vi "data read.vi"(8 "error in (no error)":errorcluster, 9 "新元素/子数组":u32, 10 "Array":u8[](array[numeric]), 11 "connection ID":refnum<k5>) -> (0 "error out":errorcluster, 1 "connection ID 2":refnum<k5>, 2 "数组 2":i32[][](array[numeric]), 3 "SEU number":u32)   [LabVIEW 2015]
panel:
  out "布尔":bool
  out "SEU？":bool
  in  "行":u32
  in  "停止":bool
  out "数据输出":string
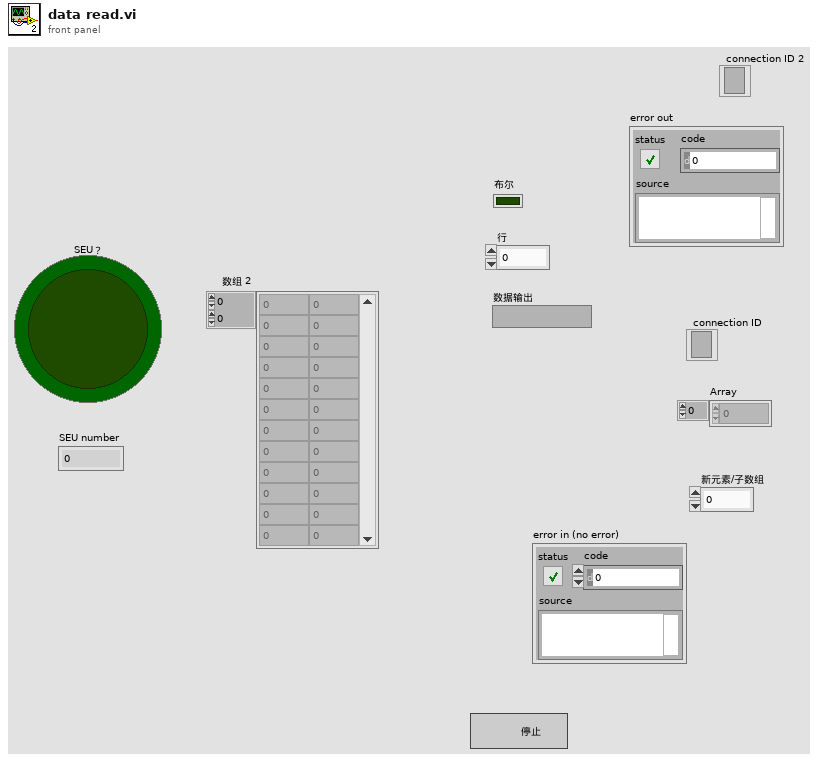
[diagram p1: front panel]
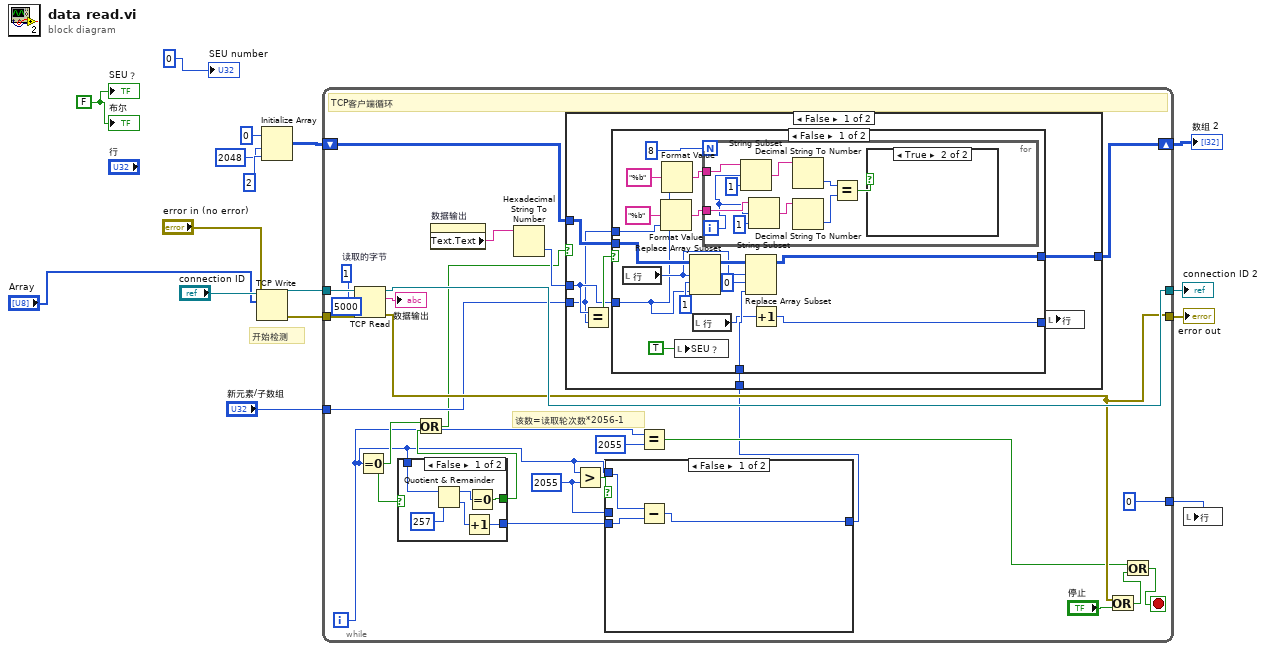
[diagram p0: block diagram]
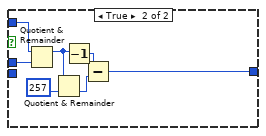
[diagram p2: hidden frame]
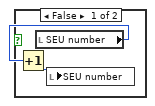
[diagram p3: hidden frame]
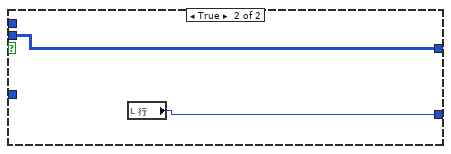
[diagram p4: hidden frame]
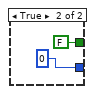
[diagram p6: hidden frame]
diagram:
  w9 = FALSE ("布尔")
  # "开始检测"
  n1 = TCP Write(connection ID="connection ID", data in="Array", error in (no error)="error in (no error)") -> (connection ID out=w15:refnum<k5>, error out=w16:errorcluster)  [unwired: 1 in, 1 out]
  n2 = Initialize Array(0 ("元素"), 2048 ("维数大小"), 2 ("维数大小")) -> (w11:i32[][])
  n3 = while {
    tunnel: w16 -> [w41]
    tunnel: w15 -> [w42]
    tunnel: [w38] -> w2
    tunnel: [w37] -> w1
    tunnel: "新元素/子数组" -> [w30]
    shift-right: [w23] -> w8
    shift-left: w11 -> [w26]
    tunnel: [u32 0 ("行")] -> w10
    i -> [w21]
    stop <- w34 stop-if-true
    w24 = 2055 ("y")
    w40 = 1  # 读取的字节
    # "该数=读取轮次数*2056-1"
    # "TCP客户端循环"
    n4 = TCP Read(connection ID=w42, bytes to read=w40, error in (no error)=w41, 9:5000 ("超时毫秒(25000)")) -> (connection ID out=w38:refnum<k5>, data out=→"数据输出":string, error out=w37:errorcluster)  [unwired: 1 in]
    n5 = Equal To 0?(x=w21) -> (x = 0?=w29:bool)
    n6 = case shown="False" w29 {
      tunnel: w21 -> [w92 _]
      tunnel: [w95 FALSE] -> w28
      tunnel: [w93 0] -> w19
      frame False {
        n7 = Quotient & Remainder(x=w92, y=257) -> (x-y*floor(x/y)=w96:i32, floor(x/y)=w94:i32)
        n8 = Increment(x=w94) -> (x+1=w93:i32)
        n9 = Equal To 0?(x=w96) -> (x = 0?=w95:bool)
      }
      frame True {
      }
    }
    n10 = Or(x=w29, y=w28) -> (x .or. y?=w27:bool)
    n11 = property on="数据输出" class="Str"() -> ("Text.Text"=w18:string)  [unwired: 2 in, 2 out]
    n12 = Hexadecimal String To Number(string=w18) -> (number=w31:u32)  [unwired: 2 in, 1 out]
    n13 = Greater?(x=w21, y=w24) -> (0:w25:bool)
    n14 = case shown="False" w25 {
      tunnel: w21 -> [w43 w52]
      tunnel: w24 -> [_ w51]
      tunnel: [w44 w47] -> w20
      tunnel: w19 -> [w45 _]
      frame False {
        n15 = Subtract(x=w43, y=w45) -> (x-y=w44:i32)
      }
      frame True {
        n16 = Quotient & Remainder(x=w52, y=w51) -> (x-y*floor(x/y)=w50:i32)  [unwired: 1 out]
        n17 = Quotient & Remainder(x=w50, y=257) -> (floor(x/y)=w48:i32)  [unwired: 1 out]
        n18 = Decrement(x=w50) -> (x-1=w46:i32)
        n19 = Subtract(x=w46, y=w48) -> (x-y=w47:i32)
      }
    }
    n20 = case shown="False" w27 {
      tunnel: w31 -> [w56 _]
      tunnel: w30 -> [w53 _]
      tunnel: w26 -> [w58 w91]
      tunnel: w20 -> [w57 _]
      tunnel: [w55 w91] -> w23
      frame False {
        n21 = Equal?(x=w56, y=w53) -> (x = y?=w59:bool)
        n22 = case shown="False" w59 {
          tunnel: w58 -> [w76 w90]
          tunnel: w57 -> [w71 _]
          tunnel: w56 -> [w64 _]
          tunnel: [w70 w90] -> w55
          tunnel: [w68 w89] -> w54
          tunnel: w53 -> [w61 _]
          frame False {
            n23 = local read "行"() -> (w73:u32)
            n24 = Format Value(format string="%b" ("格式字符串"), value (0)=w61) -> (output string=w60:string)  [unwired: 1 in]
            n25 = Format Value(format string="%b" ("格式字符串"), value (0)=w64) -> (output string=w63:string)  [unwired: 1 in]
            n26 = local write "SEU？"(TRUE ("SEU？")) -> ()
            n27 = Replace Array Subset(array=w76, new element=w64, index (row)=w73, index (col)=1 ("禁用的索引 (列)")) -> (w74:i32[][])
            n28 = local read "行"() -> (w69:u32)
            n29 = for {
              N: 8 -> [_]
              tunnel: w63 -> [w86]
              tunnel: w60 -> [w82]
              i -> [w81]
              n30 = String Subset(string=w86, offset (0)=w81, length (rest)=1 ("长度（剩余）")) -> (substring=w84:string)
              n31 = String Subset(string=w82, offset (0)=w81, length (rest)=1 ("长度（剩余）")) -> (substring=w80:string)
              n32 = Decimal String To Number(string=w84) -> (number=w79:i32)  [unwired: 2 in, 1 out]
              n33 = Decimal String To Number(string=w80) -> (number=w78:i32)  [unwired: 2 in, 1 out]
              n34 = Equal?(x=w79, y=w78) -> (x = y?=w77:bool)
              n35 = case shown="True" w77 {
                frame False {
                  n36 = local read "SEU number"() -> (w88:u32)
                  n37 = Increment(x=w88) -> (x+1=w87:u32)
                  n38 = local write "SEU number"(w87) -> ()
                }
                frame True {
                }
              }
            }
            n39 = Replace Array Subset(array=w74, new element=w71, index (row)=w73, index (col)=0 ("禁用的索引 (列)")) -> (w70:i32[][])
            n40 = Increment(x=w69) -> (x+1=w68:u32)
          }
          frame True {
            n41 = local read "行"() -> (w89:u32)
          }
        }
        n42 = local write "行"(w54) -> ()
      }
      frame True {
      }
    }
    n43 = Equal?(x=w21, y=2055) -> (x = y?=w36:bool)
    n44 = Or(x=w37, y="停止") -> (x .or. y?=w35:bool)
    n45 = Or(x=w36, y=w35) -> (x .or. y?=w34:bool)
  }
  "数组 2" <- w8
  "connection ID 2" <- w2
  "error out" <- w1
  n46 = local write "行"(w10) -> ()
  "SEU？" <- w9
  "布尔" <- w9
  "SEU number" <- u32 0 ("SEU number")
